vi "Read (Multiple Waveforms).vi"(8 "error in (no error)":errorcluster, 9 "Timeout (10000 ms)":u32=10000, 10 "Channels":u16[](array[ring]) items=["Channel 1", "Channel 2", "Channel 3", "Channel 4", "Math", "Reference A", "Reference B", "Reference C", "Reference D", "FFT"], 11 "VISA resource name":refnum<visa-resource-name>) -> (0 "error out":errorcluster, 2 "Waveform Data":waveform(dbl)[](graph), 3 "VISA resource name out":refnum<visa-resource-name>)   [LabVIEW 2017, in "Tektronix TDS 200 1000 2000 Series.lvlib"]
doc: "Initiates an acquisition on all channels that you enabled with the <B>Configure Channel</B> VI. The VI waits for the acquisition to complete and returns the waveform for the <B>Source Channels</B> you specified. If the oscilloscope did not complete the acquisition within the time period you specify with the Timeout parameter, the VI returns a timeout error. A common cause for a timeout error is the acquisition was not triggered. For example, the trigger level is out of range of the waveform. \n\n<b>Note(s):</b>\nIf your instrument does not support auto compensation for probe attenuation, you may need to adjust the scaling of the Waveform Data accordingly. This is handled automatically in the <B>Configure Channel</B> VI or can be done manually by multiplying the Waveform Data by the probe attenuation."
uses:
  Tektronix TDS 200 1000 2000 Series.lvlib
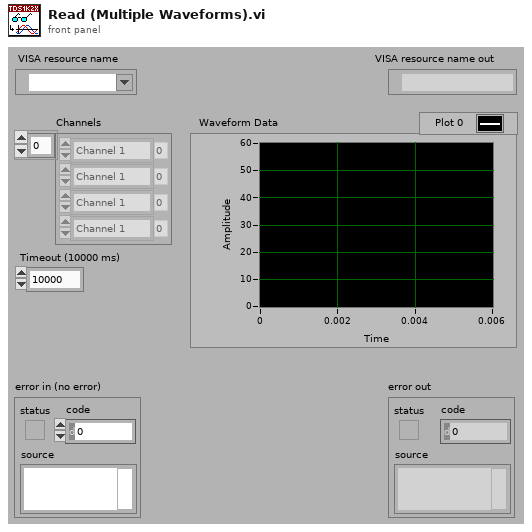
[diagram p1: front panel]
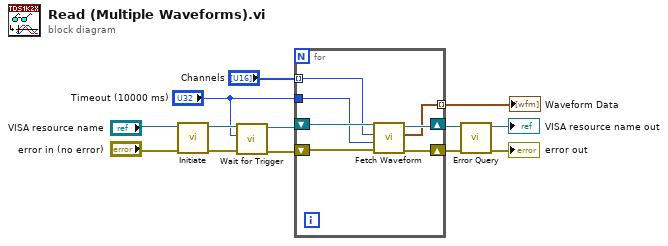
[diagram p0: block diagram]
diagram:
  n1 = call "Initiate.vi"("error in (no error)"="error in (no error)", "VISA resource name"="VISA resource name") -> ("error out"=w2:errorcluster, "VISA resource name out"=w5:refnum<visa-resource-name>)  [unwired: 8 out]
  n2 = call "Wait for Trigger.vi"("error in (no error)"=w2, "Timeout (10000 ms)"="Timeout (10000 ms)", "VISA resource name"=w5) -> ("error out"=w3:errorcluster, "VISA resource name out"=w4:refnum<visa-resource-name>)  [unwired: 7 out]
  n3 = for {
    shift-right: [w19] -> w10
    shift-left: w3 -> [w17]
    tunnel: "Channels" -> [w14] mode=indexing
    tunnel: [w16] -> w6 mode=indexing
    tunnel: "Timeout (10000 ms)" -> [w15]
    shift-right: [w20] -> w11
    shift-left: w4 -> [w18]
    n4 = call "Fetch Waveform.vi"("error in (no error)"=w17, "Timeout (10000 ms)"=w15, "Source (0: Channel 1)"=w14, "VISA resource name"=w18) -> ("error out"=w19:errorcluster, "Waveform Data"=w16:waveform(dbl), "VISA resource name out"=w20:refnum<visa-resource-name>)  [unwired: 2 in, 3 out]
  }
  "Waveform Data" <- w6
  n5 = call "Error Query.vi"("error in (no error)"=w10, "VISA resource name"=w11) -> ("error out"=→"error out":errorcluster, "VISA resource name out"=→"VISA resource name out":refnum<visa-resource-name>)  [unwired: 8 out]
